vi "Main.vi"() -> ()   [LabVIEW 2016]
doc: "The myRIO Project template acquires acceleration data from the onboard accelerometer and displays the changes of acceleration values in a waveform chart."
uses:
  <vilib>/myRIO/Instrument Drivers/Onboard IO/DIO/typedefs/DIO Reference.ctl
  <vilib>/myRIO/Common/Instrument Driver Framework/Utilities/typedefs/myRIO Generic Hardware Reference.ctl
  <vilib>/myRIO/Common/Instrument Driver Framework/Utilities/typedefs/Hardware Version Enum.ctl
  <vilib>/myRIO/Common/Instrument Driver Framework/Utilities/typedefs/myRIO v1.0 Reference.ctl
  <vilib>/myRIO/Common/Instrument Driver Framework/Utilities/typedefs/Generic FPGA Reference.ctl
  <vilib>/myRIO/Common/Instrument Driver Framework/myRIO v1.0/DIO/typedefs/DIO Channels List.ctl
  <vilib>/myRIO/Common/Instrument Driver Framework/myRIO v1.0/DIO/typedefs/DIO Channels Enum.ctl
  <vilib>/userdefined/High Color/nirio_resource_hc.ctl
  <vilib>/myRIO/Common/Instrument Driver Framework/Utilities/vis/Is FPGA Ref Available.vi
  <vilib>/myRIO/Common/Instrument Driver Framework/myRIO v1.0/DIO/vis/myRIO v1.1 Open DIO.vi
  <vilib>/myRIO/Instrument Drivers/Onboard IO/DIO/vis/Write.vi
  <vilib>/myRIO/Instrument Drivers/Onboard IO/DIO/vis/Read.vi
  <vilib>/myRIO/Common/Instrument Driver Framework/Utilities/vis/Validate Channels.vi
  <vilib>/myRIO/Common/Instrument Driver Framework/myRIO v1.0/DIO/vis/myRIO v1.0 Reserve DIO.vi
  <vilib>/myRIO/Common/Instrument Driver Framework/myRIO v1.0/UART/vis/myRIO v1.0 Close UART.vi
  <vilib>/myRIO/Common/Instrument Driver Framework/myRIO v1.0/Resource Manager/vis/myRIO v1.0 Reserve Channel List.vi
  <vilib>/myRIO/Common/Instrument Driver Framework/myRIO v1.0/DIO/vis/myRIO v1.0 Build MUX Configuration DIO.vi
  <vilib>/myRIO/Common/Instrument Driver Framework/myRIO v1.0/Resource Manager/vis/myRIO v1.0 Reserve Channel.vi
  <vilib>/myRIO/Common/Instrument Driver Framework/myRIO v1.0/Resource Manager/vis/myRIO v1.0 Unreserve Channel.vi
  <vilib>/myRIO/Common/Instrument Driver Framework/myRIO v1.0/Resource Manager/vis/myRIO v1.0 Create Configuration List.vi
  <vilib>/myRIO/Common/Instrument Driver Framework/myRIO v1.0/Resource Manager/vis/myRIO v1.0 Build Mutex Name.vi
  <vilib>/Utility/VariantDataType/GetNumericInfo.vi
  <vilib>/Utility/error.llb/Error Cluster From Error Code.vi
  <vilib>/myRIO/Common/Instrument Driver Framework/myRIO v1.0/myRIO v1.1 Open.vi
  <vilib>/myRIO/Common/Instrument Driver Framework/Utilities/vis/IO Manager.vi
  <vilib>/myRIO/Common/Instrument Driver Framework/Utilities/vis/Configuration Manager.vi
  <vilib>/myRIO/Common/Instrument Driver Framework/myRIO v1.0/Resource Manager/vis/myRIO v1.0 Configure IO.vi
  <vilib>/myRIO/Common/Instrument Driver Framework/myRIO v1.0/myRIO v1.0 Close.vi
  <vilib>/myRIO/Common/Instrument Driver Framework/myRIO v1.0/DIO/vis/myRIO v1.0 Write DIO.vi
  <vilib>/myRIO/Common/Instrument Driver Framework/myRIO v1.0/DIO/vis/myRIO v1.0 Read DIO.vi
  <vilib>/myRIO/Common/Instrument Driver Framework/Utilities/vis/FPGA Ref Manager.vi
  <vilib>/myRIO/Common/Instrument Driver Framework/myRIO v1.0/myRIO v1.0 Reset FPGA.vi
  <vilib>/myRIO/Common/Instrument Driver Framework/myRIO v1.0/IRQ/vis/myRIO v1.0 IRQ Info FGV.vi
  <vilib>/myRIO/Common/Instrument Driver Framework/myRIO v1.0/IRQ/vis/myRIO v1.0 Timer IRQ Info FGV.vi
  <vilib>/myRIO/Common/Instrument Driver Framework/myRIO v1.0/IRQ/vis/myRIO v1.0 ISR Agent.vi
  <vilib>/myRIO/Express VI/Onboard IO/DO/DO Express VI.xnode
  <vilib>/myRIO/Instrument Drivers/Onboard IO/DIO/vis/myRIO DIO Open.xnode
  <vilib>/myRIO/Express VI/Onboard IO/DI/DI Express VI.xnode
  <vilib>/myRIO/Instrument Drivers/Onboard IO/DIO/DIO.lvlib
  <vilib>/myRIO/Instrument Drivers/Utilities/Utilities.lvlib
panel:
  out "error out":errorcluster
  in  "Stop":bool
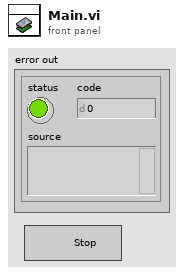
[diagram p1: front panel]
types:
  T1 = typedef "DIO.lvlib/DIO Reference.ctl" = cluster{"myRIO Reference":T2, "DIO Channels List":T6}
  T2 = typedef "myRIO Generic Hardware Reference.ctl" = cluster{"myRIO Model":T3, "myRIO Hardware Reference":T4}
  T3 = typedef "Hardware Version Enum.ctl" = enum16{"Unknown", "myRIO-1900", "myRIO-1950", "roboRIO", "NI ELVIS RIO CM"}
  T4 = typedef "myRIO v1.0 Reference.ctl" = cluster{"Generic FPGA Reference":T5, "Allow multiple opens":bool}
  T5 = typedef "Generic FPGA Reference.ctl" = refnum<k20>
  T6 = typedef "DIO Channels List.ctl" = T7[]
  T7 = typedef "DIO Channels Enum.ctl" = enum16{"Not Connected", "C/DIO0", "C/DIO1", "C/DIO2", "C/DIO3", "C/DIO4", "C/DIO5", "C/DIO6", "C/DIO7", "A/DIO0", "A/DIO1", "A/DIO2", "A/DIO3", "A/DIO4", "A/DIO5", "A/DIO6", "A/DIO7", "A/DIO8", "A/DIO9", "A/DIO10", "A/DIO11", "A/DIO12", "A/DIO13", "A/DIO14", "A/DIO15", "B/DIO0", "B/DIO1", "B/DIO2", "B/DIO3", "B/DIO4", "B/DIO5", "B/DIO6", "B/DIO7", "B/DIO8", "B/DIO9", "B/DIO10", "B/DIO11", "B/DIO12", "B/DIO13", "B/DIO14", "B/DIO15", "LED0", "LED1", "LED2", "LED3", "Button0", "DIO/DIO0", "DIO/DIO1", "DIO/DIO2", "DIO/DIO3", "DIO/DIO4", "DIO/DIO5", "DIO/DIO6", "DIO/DIO7", "DIO/DIO8", "DIO/DIO9", "SPI/CS0", "SPI/CS1", "SPI/CS2", "SPI/CS3", "LED RADIO (Green)", "LED RADIO (Red)", "LED COMM (Green)", "LED COMM (Red)", "LED MODE (Green)", "LED MODE (Red)"}
  T8 = typedef "nirio_resource_hc.ctl" = tag
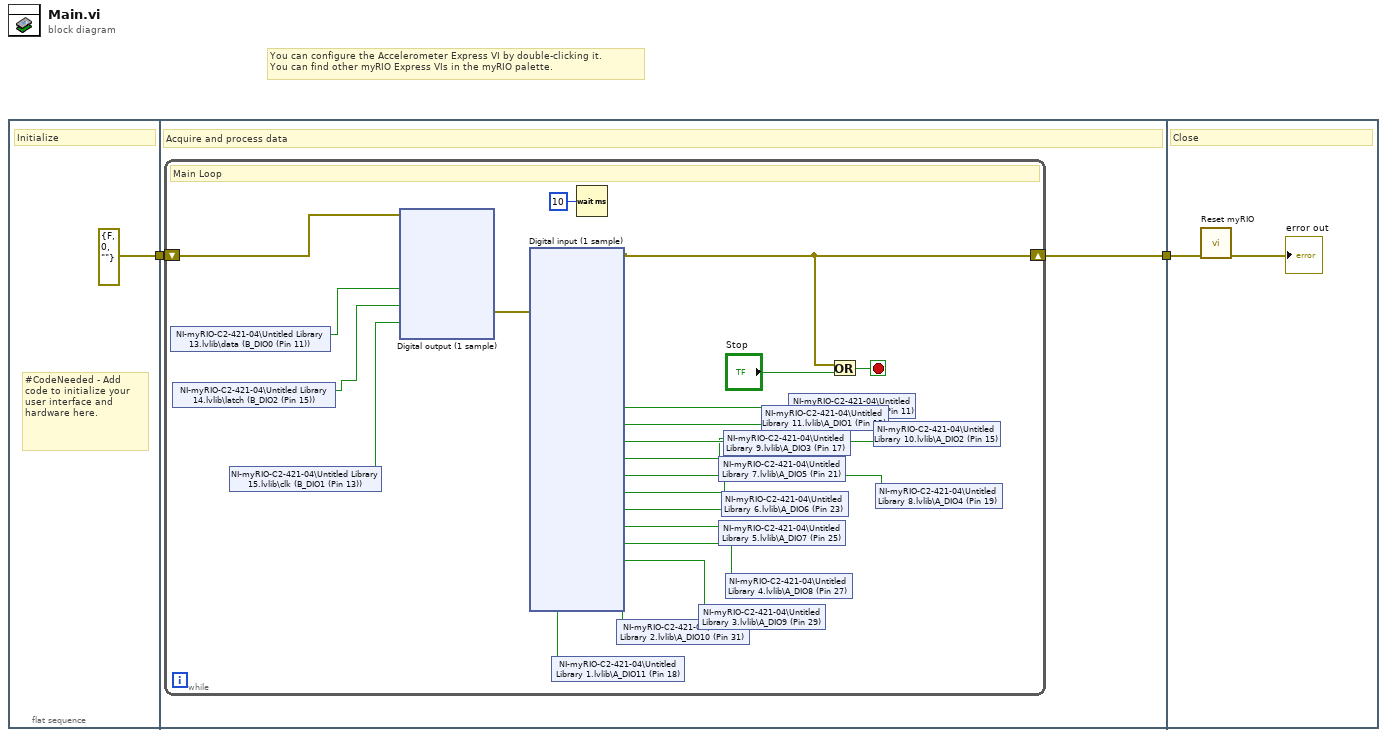
[diagram p0: block diagram]
diagram:
  # "You can configure the Accelerometer Express VI by double-clicking it.\nYou can find other myRIO Express VIs in the myRIO palette."
  n1 = flat-sequence {
    tunnel: [errorcluster {"status"=FALSE, "code"=0, "source"=""} ("error in (no error)")] -> w2
    tunnel: w2 -> [w5]
    tunnel: [w4] -> w1
    tunnel: w1 -> [w111]
    frame #0 {
      # "#CodeNeeded - Add code to initialize your user interface and hardware here."
      # "Initialize"
    }
    frame #1 {
      # "Acquire and process data"
      n2 = while {
        shift-right: [w23] -> w4
        shift-left: w5 -> [w21]
        stop <- w25 stop-if-true
        # "Main Loop"
        n3 = shared-variable "NI-myRIO-C2-421-04\\Untitled Library 13.lvlib\\data (B_DIO0 (Pin 11))"() -> (w7:bool)  [unwired: 1 in, 1 out]
        n4 = shared-variable "NI-myRIO-C2-421-04\\Untitled Library 14.lvlib\\latch (B_DIO2 (Pin 15))"() -> (w6:bool)  [unwired: 1 in, 1 out]
        n5 = shared-variable "NI-myRIO-C2-421-04\\Untitled Library 15.lvlib\\clk (B_DIO1 (Pin 13))"() -> (w8:bool)  [unwired: 1 in, 1 out]
        n6 = xnode "Digital output (1 sample)"("data (B/DIO0 (Pin 11))"=w7, "latch (B/DIO2 (Pin 15))"=w6, "clk (B/DIO1 (Pin 13))"=w8, "error in (no error)"=w21) -> ("error out"=w22:errorcluster)
        n7 = xnode "Digital input (1 sample)"("error in (no error)"=w22) -> ("A/DIO0 (Pin 11)"=w9:bool, "A/DIO1 (Pin 13)"=w10:bool, "A/DIO2 (Pin 15)"=w20:bool, "A/DIO3 (Pin 17)"=w11:bool, "A/DIO4 (Pin 19)"=w12:bool, "A/DIO5 (Pin 21)"=w19:bool, "A/DIO6 (Pin 23)"=w18:bool, "A/DIO7 (Pin 25)"=w17:bool, "A/DIO8 (Pin 27)"=w16:bool, "A/DIO9 (Pin 29)"=w15:bool, "A/DIO10 (Pin 31)"=w14:bool, "A/DIO11 (Pin 18)"=w13:bool, "error out"=w23:errorcluster)
        n8 = shared-variable "NI-myRIO-C2-421-04\\Untitled Library 1.lvlib\\A_DIO11 (Pin 18)"(w13) -> ()  [unwired: 1 in, 1 out]
        n9 = Wait (ms)(milliseconds to wait=u32 10) -> ()  [unwired: 1 out]
        n10 = shared-variable "NI-myRIO-C2-421-04\\Untitled Library 2.lvlib\\A_DIO10 (Pin 31)"(w14) -> ()  [unwired: 1 in, 1 out]
        n11 = shared-variable "NI-myRIO-C2-421-04\\Untitled Library 3.lvlib\\A_DIO9 (Pin 29)"(w15) -> ()  [unwired: 1 in, 1 out]
        n12 = shared-variable "NI-myRIO-C2-421-04\\Untitled Library 7.lvlib\\A_DIO5 (Pin 21)"(w19) -> ()  [unwired: 1 in, 1 out]
        n13 = shared-variable "NI-myRIO-C2-421-04\\Untitled Library 5.lvlib\\A_DIO7 (Pin 25)"(w17) -> ()  [unwired: 1 in, 1 out]
        n14 = shared-variable "NI-myRIO-C2-421-04\\Untitled Library 6.lvlib\\A_DIO6 (Pin 23)"(w18) -> ()  [unwired: 1 in, 1 out]
        n15 = shared-variable "NI-myRIO-C2-421-04\\Untitled Library 9.lvlib\\A_DIO3 (Pin 17)"(w11) -> ()  [unwired: 1 in, 1 out]
        n16 = shared-variable "NI-myRIO-C2-421-04\\Untitled Library 4.lvlib\\A_DIO8 (Pin 27)"(w16) -> ()  [unwired: 1 in, 1 out]
        n17 = shared-variable "NI-myRIO-C2-421-04\\Untitled Library 11.lvlib\\A_DIO1 (Pin 13)"(w10) -> ()  [unwired: 1 in, 1 out]
        n18 = shared-variable "NI-myRIO-C2-421-04\\Untitled Library 12.lvlib\\A_DIO0 (Pin 11)"(w9) -> ()  [unwired: 1 in, 1 out]
        n19 = Or(x=w23, y="Stop") -> (x .or. y?=w25:bool)
        n20 = shared-variable "NI-myRIO-C2-421-04\\Untitled Library 10.lvlib\\A_DIO2 (Pin 15)"(w20) -> ()  [unwired: 1 in, 1 out]
        n21 = shared-variable "NI-myRIO-C2-421-04\\Untitled Library 8.lvlib\\A_DIO4 (Pin 19)"(w12) -> ()  [unwired: 1 in, 1 out]
      }
    }
    frame #2 {
      # "Close"
      n22 = call <vilib>:"Reset myRIO.vi"("error in (no error)"=w111) -> ("error out"=→"error out":errorcluster)  [unwired: 10 in]
    }
  }
